vi "故障码字段定义.vi"(7 "id":u16, 11 "故障代码":u16) -> (3 "报警":T1)   [LabVIEW 2016, in "斯坦道总磷总氮V2.lvlib"]
uses:
  Alarm interface/Alarm interface.lvlib
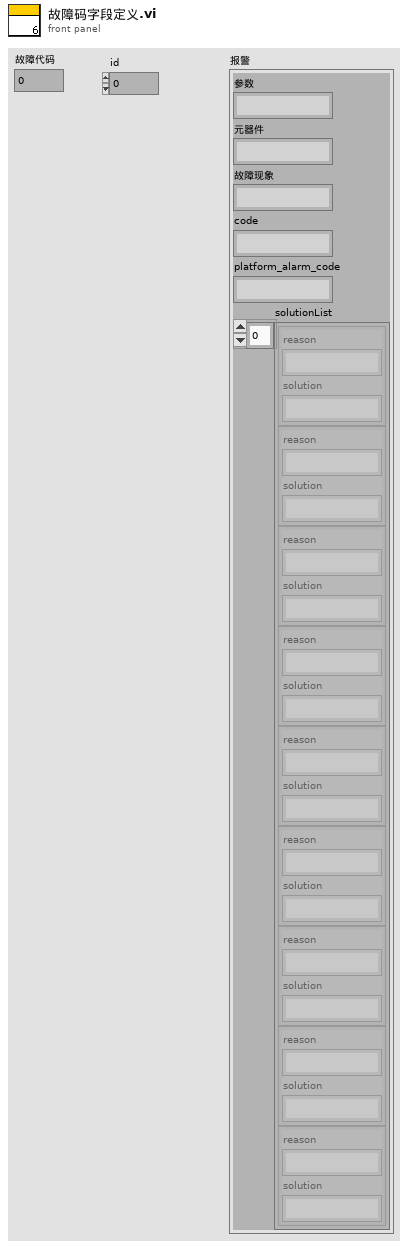
[diagram p1: front panel]
types:
  T1 = typedef "Alarm interface.lvlib/报警短信语音交互.ctl" = cluster{"参数":string, "元器件":string, "故障现象":string, "code":string, "platform_alarm_code":string, "solutionList":cluster{"reason":string, "solution":string}[]}
  T2 = typedef "Alarm interface.lvlib/map in.ctl" = cluster{"name":string, "CN":string, "FirmwareVersion":string, "code":string}
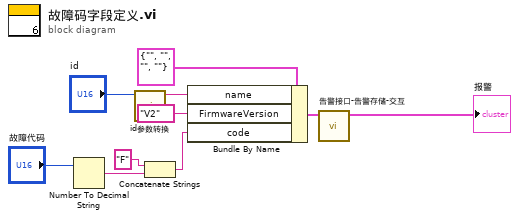
[diagram p0: block diagram]
diagram:
  n1 = Number To Decimal String(number="故障代码") -> (decimal integer string=w5:string)  [unwired: 1 in]
  n2 = call "id参数转换.vi"("id"="id") -> ("table输出"=w10:string)  [unwired: 9 in, 1 out]
  n3 = Concatenate Strings("F" ("字符串"), w5) -> (w3:string)
  n4 = Bundle By Name(cluster=T2 {"name"="", "CN"="", "FirmwareVersion"="", "code"=""} ("map in"), "name"=w10, "FirmwareVersion"="V2" ("equipVersion"), "code"=w3) -> (w1:T2)
  n5 = call "告警接口-告警存储-交互.vi"("map in"=w1) -> ("data"=→"报警":T1)  [unwired: 10 in]
